vi "update_exp_time.vi"(8 "error in":errorcluster) -> (0 "error out":errorcluster, 3 "double precision float":dbl)   [LabVIEW 2013]
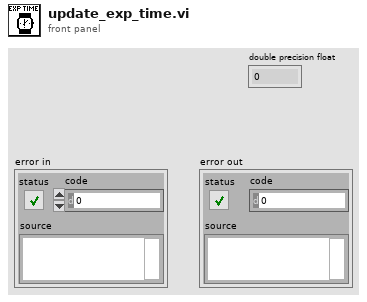
[diagram p1: front panel]
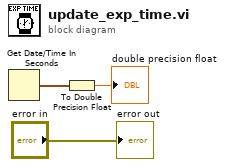
[diagram p0: block diagram]
diagram:
  n1 = Get Date/Time In Seconds() -> (seconds since 1Jan1904=w2:timestamp)
  n2 = To Double Precision Float(number=w2) -> (double precision float=→"double precision float":dbl)
  "error out" <- "error in"
